vi "题目5.vi"() -> ()   [LabVIEW 2017]
panel:
  out "日期/时间字符串":string
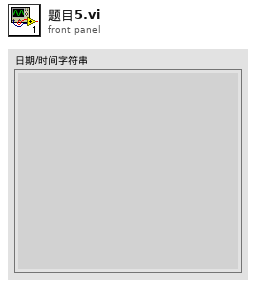
[diagram p1: front panel]
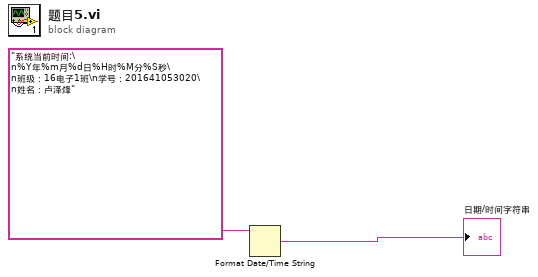
[diagram p0: block diagram]
diagram:
  n1 = Format Date/Time String(time format string (%c)="系统当前时间:\n%Y年%m月%d日%H时%M分%S秒\n班级：16电子1班\n学号：201641053020\n姓名：卢泽烽" ("时间格式字符串(%c)")) -> (date/time string=→"日期/时间字符串":string)  [unwired: 2 in]
